vi "EventPassState.vi"(10 "IA State Input":T1) -> (1 "Id":dbl, 2 "IA State Output":T1, 3 "Pass State":bool)   [LabVIEW 2016]
uses:
  Core/AI Input.ctl
  Core/AI Robot.ctl
  Intel/Functions Enum.ctl
  Intel/AttackerStates.ctl
  Core/AI Ball.ctl
  Core/Field Size.ctl
  Core/AI Judge.ctl
  Intel/Command Enum.ctl
  Events.ctl
panel:
  in  "Desabilita passe":bool=TRUE
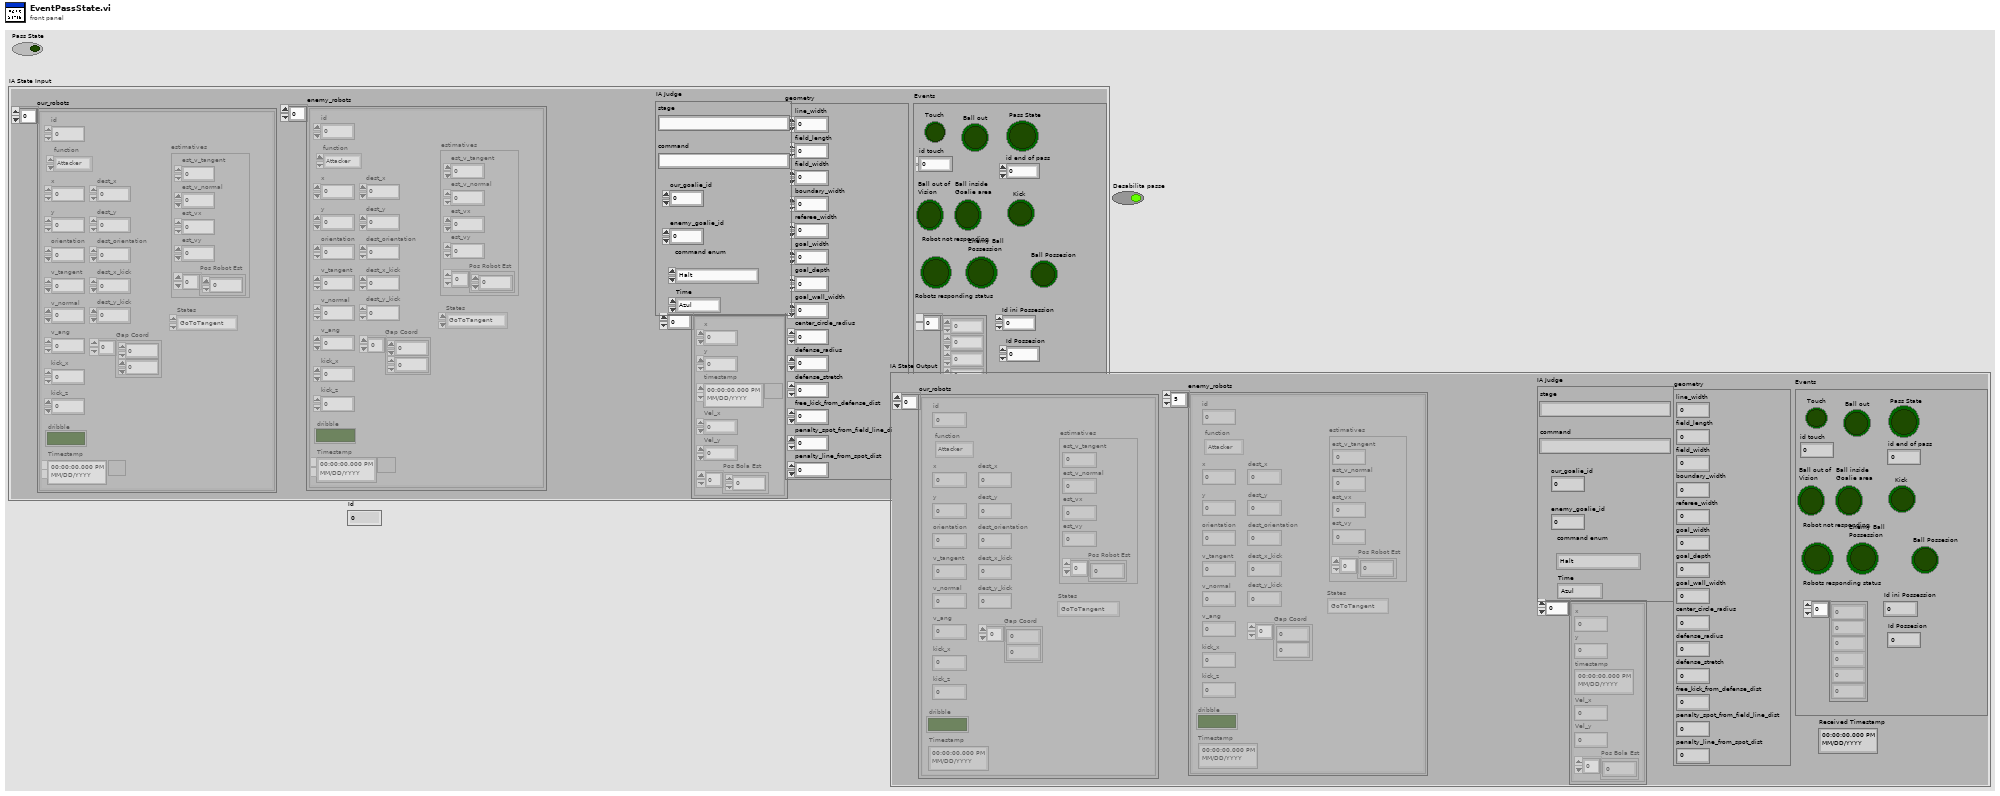
[diagram p1: front panel]
types:
  T1 = typedef "AI Input.ctl" = cluster{"our_robots":T2[], "enemy_robots":T2[], "balls":T5[], "geometry":T6, "IA Judge":T7, "Received Timestamp":timestamp, "Events":T9}
  T2 = typedef "AI Robot.ctl" = cluster{"id":u32, "function":T3, "x":dbl, "y":dbl, "orientation":dbl, "v_tangent":dbl, "v_normal":dbl, "v_ang":dbl, "kick_x":dbl, "kick_z":dbl, "dribble":bool, "Timestamp":timestamp, "dest_x":dbl, "dest_y":dbl, "dest_orientation":dbl, "estimatives":cluster{"est_v_tangent":dbl, "est_v_normal":dbl, "est_vx":dbl, "est_vy":dbl, "Pos Robot Est":dbl[]}, "dest_x_kick":dbl, "dest_y_kick":dbl, "Gap Coord":dbl[], "States":T4}
  T3 = typedef "Functions Enum.ctl" = enum16{"Attacker", "Goalie", "Defender", "Striker", "Goto 0", "Dummy", "Kicker", "ZigZag"}
  T4 = typedef "AttackerStates.ctl" = enum16{"Pass", "GoToTangent", "BallGetting", "GoToKick", ""}
  T5 = typedef "AI Ball.ctl" = cluster{"x":dbl, "y":dbl, "timestamp":timestamp, "Vel_x":dbl, "Vel_y":dbl, "Pos Bola Est":dbl[]}
  T6 = typedef "Field Size.ctl" = cluster{"line_width":u32, "field_length":u32, "field_width":u32, "boundary_width":u32, "referee_width":u32, "goal_width":u32, "goal_depth":u32, "goal_wall_width":u32, "center_circle_radius":u32, "defense_radius":u32, "defense_stretch":u32, "free_kick_from_defense_dist":u32, "penalty_spot_from_field_line_dist":u32, "penalty_line_from_spot_dist":u32}
  T7 = typedef "AI Judge.ctl" = cluster{"stage":string, "command":string, "our_goalie_id":dbl, "enemy_goalie_id":dbl, "command enum":T8, "Time":enum16{"Azul", "Amarelo"}}
  T8 = typedef "Command Enum.ctl" = enum16{"Halt", "Stop", "Force Start", "PKA Normal Start", "Prepare Kickoff Ally", "PKE Normal Start", "Prepare Kickoff Enemy", "Prepare Penalty Ally", "PPA Normal Start", "Prepare Penalty Enemy", "PPE Normal Start", "Direct Free Enemy", "Direct Free Ally", "Indirect Free Enemy", "Indirect Free Ally", "Timeout Enemy", "Timeout Ally", "Goal Enemy", "Goal Ally", "Ball Placement Enemy", "Ball Placement Ally", "Normal Half Time", "Extra Time Break", "Extra Half Time", "None", "Post Game"}
  T9 = typedef "Events.ctl" = cluster{"Touch":bool, "Ball out":bool, "id touch":dbl, "Ball out of \nVision":bool, "Ball inside \nGoalie area":bool, "Robot not responding":bool, "Robots responding status":dbl[], "Enemy Ball \nPossession":bool, "Pass State":bool, "id end of pass":dbl, "Kick":bool, "Id ini Possession":dbl, "Ball Possesion":bool, "Id Possesion":dbl}
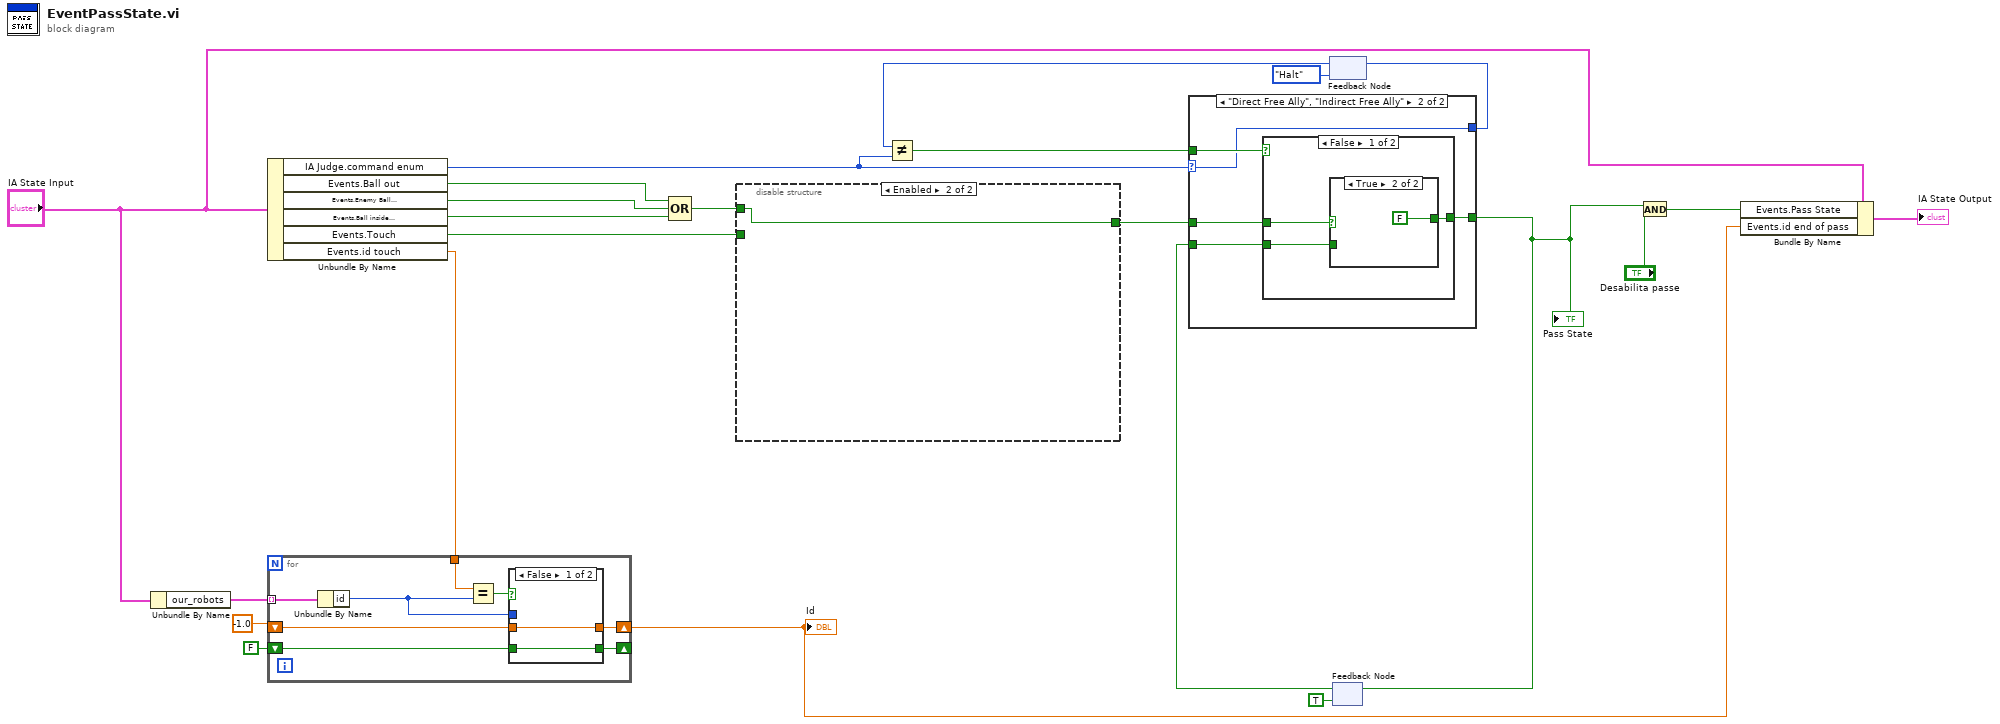
[diagram p0: block diagram]
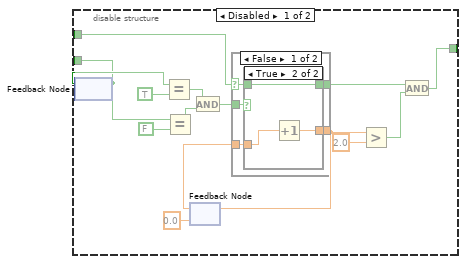
[diagram p2: hidden frame]
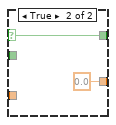
[diagram p4: hidden frame]
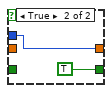
[diagram p5: hidden frame]
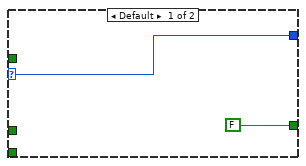
[diagram p6: hidden frame]
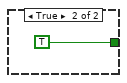
[diagram p8: hidden frame]
diagram:
  n1 = Unbundle By Name("IA State Input") -> ("our_robots"=w16:T2[])
  n2 = Unbundle By Name("IA State Input") -> ("IA Judge.command enum"=w23:T8, "Events.Ball out"=w8:bool, "Events.Enemy Ball \nPossession"=w7:bool, "Events.Ball inside \nGoalie area"=w6:bool, "Events.Touch"=w9:bool, "Events.id touch"=w15:dbl)
  n3 = for {
    tunnel: w16 -> [w31] mode=indexing
    shift-right: [w28] -> _
    shift-left: FALSE -> [w29]
    tunnel: w15 -> [w30]
    shift-right: [w25] -> w10
    shift-left: -1.0 -> [w24]
    n4 = Unbundle By Name(w31) -> ("id"=w26:u32)
    n5 = Equal?(x=w30, y=w26) -> (x = y?=w27:bool)
    n6 = case shown="False" w27 {
      tunnel: w29 -> [w33 _]
      tunnel: [w33 TRUE] -> w28
      tunnel: w26 -> [_ w34]
      tunnel: [w32 w34] -> w25
      tunnel: w24 -> [w32 _]
      frame False {
      }
      frame True {
      }
    }
  }
  "Id" <- w10
  n7 = Compound Arithmetic op=OR(w8, w7, w6) -> (w5:bool)
  n8 = disable-structure shown="Enabled" {
    disable-tunnel: w9 -> [w49 _]
    disable-tunnel: w5 -> [w39 w63]
    disable-tunnel: [w36 w63] -> w4
    frame Disabled {
      n9 = feedback #1() -> (w50:bool)  [unwired: 1 in]
      n10 = feedback-in #1(w49) -> ()
      n11 = Equal?(x=w50, y=TRUE) -> (x = y?=w46:bool)
      n12 = Equal?(x=w49, y=FALSE) -> (x = y?=w45:bool)
      n13 = feedback #2(0.0) -> (w43:dbl)
      n14 = And(x=w46, y=w45) -> (x .and. y?=w44:bool)
      n15 = case shown="False" w39 {
        selector: w39 -> [w52 w61]
        tunnel: w44 -> [w55 _]
        tunnel: w43 -> [w54 _]
        tunnel: [w53 0.0] -> w41
        tunnel: [w51 w61] -> w37
        frame False {
          n16 = case shown="True" w55 {
            tunnel: [w57 w60] -> w53
            tunnel: w54 -> [w57 w59]
            tunnel: w52 -> [w56 w58]
            tunnel: [w56 w58] -> w51
            frame False {
            }
            frame True {
              n17 = Increment(x=w59) -> (x+1=w60:dbl)
            }
          }
        }
        frame True {
        }
      }
      n18 = feedback-in #2(w41) -> ()
      n19 = Greater?(x=w41, y=2.0) -> (0:w38:bool)
      n20 = And(x=w37, y=w38) -> (x .and. y?=w36:bool)
    }
    frame Enabled {
    }
  }
  n21 = feedback #3(Command_Enum."Halt" ("command\nenum")) -> (w22:T8)
  n22 = Not Equal?(x=w22, y=w23) -> (x != y?=w21:bool)
  n23 = feedback #4(TRUE) -> (w20:bool)
  n24 = case shown="\"Direct Free Ally\", \"Indirect Free Ally\"" w23 {
    selector: w23 -> [w64 w66]
    tunnel: w4 -> [_ w70]
    tunnel: w21 -> [_ w69]
    tunnel: [FALSE w68] -> w3
    tunnel: w20 -> [_ w67]
    tunnel: [w64 w66] -> w19
    frame Default {
    }
    frame "Direct Free Ally", "Indirect Free Ally" {
      n25 = case shown="False" w69 {
        tunnel: w70 -> [w73 _]
        tunnel: [w72 TRUE] -> w68
        tunnel: w67 -> [w71 _]
        frame False {
          n26 = case shown="True" w73 {
            tunnel: [w74 FALSE] -> w72
            tunnel: w71 -> [w74 _]
            frame False {
            }
            frame True {
            }
          }
        }
        frame True {
        }
      }
    }
  }
  "Pass State" <- w3
  n27 = feedback-in #3(w19) -> ()
  n28 = feedback-in #4(w3) -> ()
  n29 = And(x=w3, y="Desabilita passe") -> (x .and. y?=w2:bool)
  n30 = Bundle By Name(cluster="IA State Input", "Events.Pass State"=w2, "Events.id end of pass"=w10) -> (→"IA State Output":T1)
